vi "udp_publish.vi"(8 "error in":errorcluster, 11 "UDP Publisher":T2={"UDP Configuration"={"connection ID"=refnum, "Local"={"Port "=10100, "Timeout (ms)"=5000}, "Destination"={"IP Address"="192.168.1.10", "Port "=5016, "Timeout (ms)"=5000}}, "Update Period [.001 secs]"=50, "error out"={"status"=FALSE, "code"=0, "source"=""}, "Stop"=FALSE, "Activity"=FALSE, "Finished\nLate?"=FALSE, "Data Transmitted"=""}) -> (0 "error out":errorcluster, 3 "UDP Publisher [out]":T2={"UDP Configuration"={"connection ID"=refnum, "Local"={"Port "=10100, "Timeout (ms)"=5000}, "Destination"={"IP Address"="192.168.1.10", "Port "=5016, "Timeout (ms)"=5000}}, "Update Period [.001 secs]"=50, "error out"={"status"=FALSE, "code"=0, "source"=""}, "Stop"=FALSE, "Activity"=FALSE, "Finished\nLate?"=FALSE, "Data Transmitted"=""})   [LabVIEW 2014]
uses:
  typedefs/udp__pub_configuration.ctl
  typedefs/udp_publisher.ctl
panel:
  in  "Tab Control":enum32{"Main Display", "I/O Controls"}(tab)
  out "Transmitted String":string
  out "UDP Configuration (out)":T1
  out "UDP Configuration (in)":T1
  # "UDP Publisher"
  # "UDP Publish:"
  # "UDP Publish:"
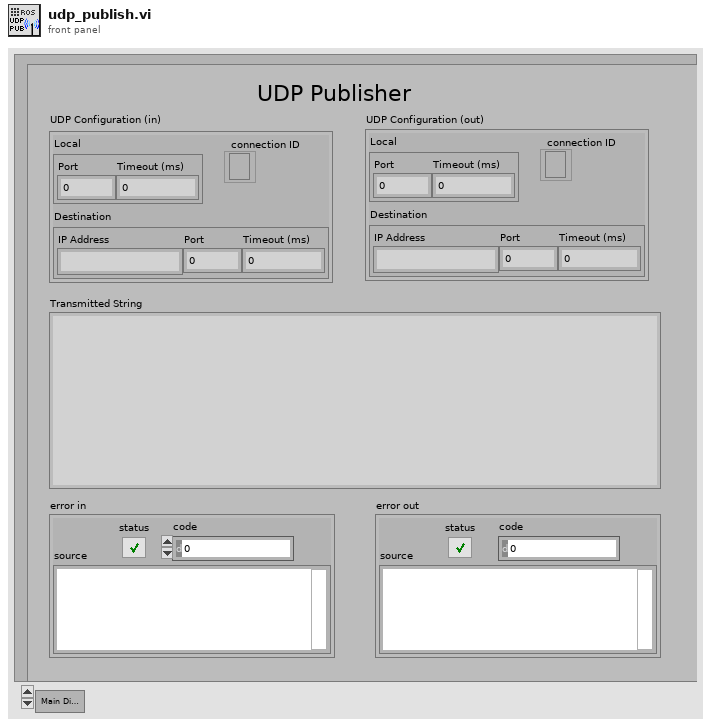
[diagram p1: front panel]
types:
  T1 = typedef "udp__pub_configuration.ctl" = cluster{"connection ID":refnum<k16>, "Local":cluster{"Port ":u16, "Timeout (ms)":i32}, "Destination":cluster{"IP Address":string, "Port ":u16, "Timeout (ms)":i32}}
  T2 = typedef "udp_publisher.ctl" = cluster{"UDP Configuration":T1, "Update Period [.001 secs]":i64, "error out":errorcluster, "Stop":bool, "Activity":bool, "Finished\nLate?":bool, "Data Transmitted":string}
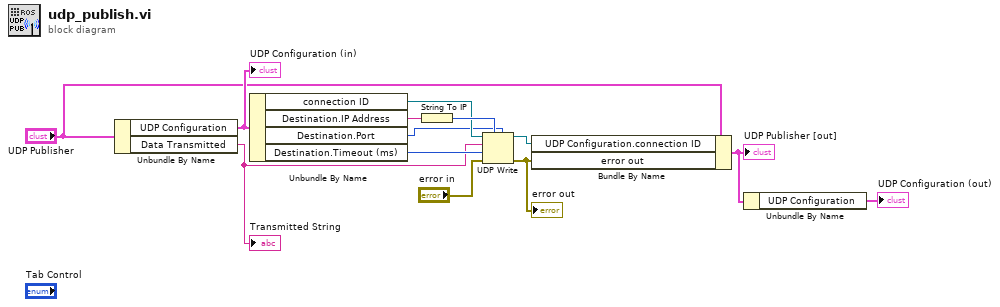
[diagram p0: block diagram]
diagram:
  n1 = Unbundle By Name("UDP Publisher") -> ("UDP Configuration"=w6:T1, "Data Transmitted"=w1:string)
  "UDP Configuration (in)" <- w6
  "Transmitted String" <- w1
  n2 = Unbundle By Name(w6) -> ("connection ID"=w12:refnum<k16>, "Destination.IP Address"=w10:string, "Destination.Port"=w11:u16, "Destination.Timeout (ms)"=w8:i32)
  n3 = String To IP(1:w10) -> (0:w13:u32)
  n4 = UDP Write(address=w13, port or service name=w11, connection ID=w12, data in=w1, 8:"error in", 9:w8) -> (error out=w2:errorcluster, 3:w9:refnum<k16>)
  "error out" <- w2
  n5 = Bundle By Name(cluster="UDP Publisher", "UDP Configuration.connection ID"=w9, "error out"=w2) -> (w4:T2)
  "UDP Publisher [out]" <- w4
  n6 = Unbundle By Name(w4) -> ("UDP Configuration"=→"UDP Configuration (out)":T1)
